vi "array_compile.vi"(10 "dataIn":u32, 11 "ArrayIn":bool[][](array[boolean])) -> (3 "ArrayOut":bool[][](array[boolean]))   [LabVIEW 2021]
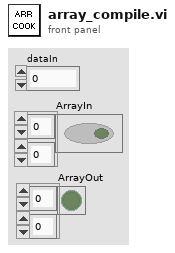
[diagram p1: front panel]
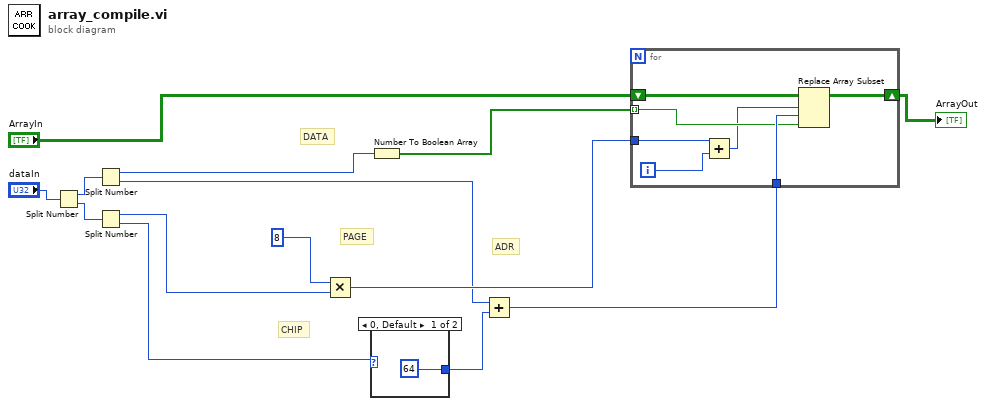
[diagram p0: block diagram]
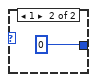
[diagram p2: hidden frame]
diagram:
  # "CHIP"
  # "PAGE"
  # "ADR"
  # "DATA"
  n1 = Split Number(x="dataIn") -> (hi(x)=w6:u16, lo(x)=w5:u16)
  n2 = Split Number(x=w6) -> (hi(x)=w4:u8, lo(x)=w3:u8)
  n3 = Split Number(x=w5) -> (hi(x)=w2:u8, lo(x)=w1:u8)
  n4 = Multiply(x=u32 8, y=w2) -> (x*y=w11:u32)
  n5 = case shown="0, Default" w1 {
    tunnel: [64 0] -> w8
    frame 0, Default {
    }
    frame 1 {
    }
  }
  n6 = Number To Boolean Array(number=w4) -> (Boolean array=w12:bool[])
  n7 = Add(x=w3, y=w8) -> (x+y=w13:i32)
  n8 = for {
    tunnel: w13 -> [w23]
    shift-right: [w21] -> w10
    shift-left: "ArrayIn" -> [w22]
    tunnel: w12 -> [w20] mode=indexing
    tunnel: w11 -> [w19]
    i -> [w18]
    n9 = Add(x=w19, y=w18) -> (x+y=w17:u32)
    n10 = Replace Array Subset(array=w22, new element=w20, index (row)=w17, index (col)=w23) -> (w21:bool[][])
  }
  "ArrayOut" <- w10
